vi "Spartan HTTP VIT Open.vi"(8 "error in":errorcluster, 9 "rendezvous":string, 10 "Parent VI Name (\"\")":string, 11 "HTTP session":T1 {"object data"."time" format="%0.2f"}) -> (0 "error out":errorcluster, 1 "content":string, 2 "env":T3, 3 "HTTP session out":T1 {"object data"."time" format="%0.2f"})   [LabVIEW 2011]
uses:
  Spartan HTTP Session.ctl
  Addons/internet/http/http_obj.llb/HTTP Session Data.ctl
  Addons/internet/utils/keyedarr.llb/Keyed Array.ctl
  Spartan HTTP Server Globals.vi
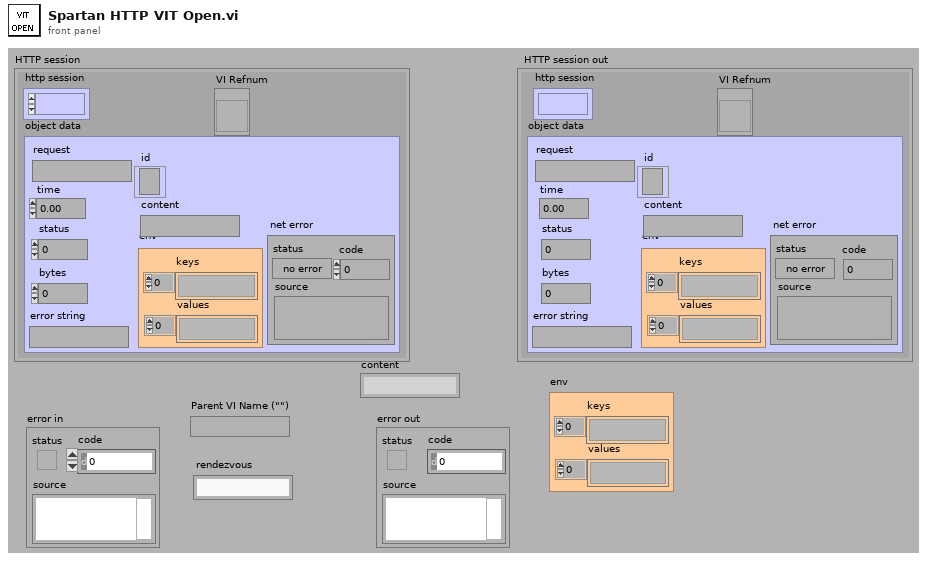
[diagram p1: front panel]
types:
  T1 = typedef "Spartan HTTP Session.ctl" = cluster{"http session":refnum<k1>, "object data":T2, "VI Refnum":refnum<vi>}
  T2 = typedef "HTTP Session Data.ctl" = cluster{"request":string, "time":dbl, "status":i32, "error string":string, "bytes":i32, "env":T3, "content":string, "id":refnum<k5>, "net error":errorcluster}
  T3 = typedef "Keyed Array.ctl" = cluster{"keys":string[], "values":string[]}
  T4 = typedef "Semaphore RefNum" = refnum<k1>
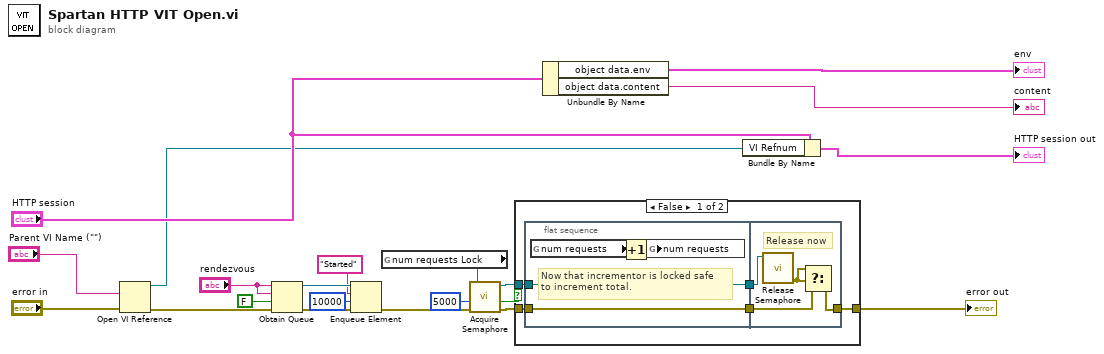
[diagram p0: block diagram]
diagram:
  n1 = Open VI Reference(vi path="Parent VI Name (\"\")", error in (no error)="error in") -> (vi reference=w17:refnum<vi>, error out=w15:errorcluster)  [unwired: 1 in, 3 out]
  n2 = Obtain Queue(name (unnamed)="rendezvous", element data type="rendezvous", create if not found? (T)=FALSE ("return existing (F)"), error in (no error)=w15) -> (queue out=w12:refnum<queue>, error out=w11:errorcluster)  [unwired: 1 in, 1 out]
  n3 = Enqueue Element(queue=w12, element="Started" ("format string"), timeout in ms (-1)=10000 ("ms timeout (-1)"), error in (no error)=w11) -> (error out=w3:errorcluster)  [unwired: 2 out]
  n4 = global read "Spartan HTTP Server Globals.vi" "num requests Lock"() -> (w8:T4)
  n5 = call <vilib>:"Acquire Semaphore.vi"("error in (no error)"=w3, "ms timeout (-1)"=5000, "semaphore"=w8) -> ("error out"=w5:errorcluster, "timed out"=w6:bool, "semaphore out"=w4:T4)  [unwired: 2 out]
  n6 = case shown="False" w6 {
    tunnel: w5 -> [w25 w35]
    tunnel: [w22 w35] -> w2
    tunnel: w4 -> [w23 _]
    frame False {
      n7 = flat-sequence {
        tunnel: [w28] -> w26
        tunnel: w25 -> [w28]
        tunnel: [w27] -> w24
        tunnel: w23 -> [w27]
        tunnel: w26 -> [w32]
        tunnel: w24 -> [w34]
        tunnel: [w31] -> w22
        frame #0 {
          # "Now that incrementor is locked safe\nto increment total."
          n8 = global read "Spartan HTTP Server Globals.vi" "num requests"() -> (w30:u32)
          n9 = Increment(x=w30) -> (x+1=w29:u32)
          n10 = global write "Spartan HTTP Server Globals.vi" "num requests"(w29) -> ()
        }
        frame #1 {
          # "Release now"
          n11 = call <vilib>:"Release Semaphore.vi"("semaphore"=w34) -> ("error out"=w33:errorcluster)  [unwired: 1 in, 5 out]
          n12 = Select(t=w33, s=w33, f=w32) -> (s? t:f=w31:errorcluster)
        }
      }
    }
    frame True {
      # "BAD THING if can't acquire semaphore"
    }
  }
  "error out" <- w2
  n13 = Unbundle By Name("HTTP session") -> ("object data.env"=→"env":T3, "object data.content"=→"content":string)
  n14 = Bundle By Name(cluster="HTTP session", "VI Refnum"=w17) -> (→"HTTP session out":T1)
